vi "Real Cholesky Factorization.vi"(0 "A":T1) -> (1 "Cholesky":T1, 2 "error":i32)   [LabVIEW 2018, in "NI_AALPro.lvlib"]
doc: "Performs Cholesky factorization on a symmetric or Hermitian positive definite matrix. Wire data to the <B>A</B> input to determine the polymorphic instance to use or manually select the instance."
uses:
  <vilib>/Analysis/NI_AALPro.lvlib
  RealMatrix.ctl
  Full Real Matrix Cholesky Factorization.vi
  <vilib>/Analysis/NI_AALBase.lvlib
  NI_Matrix.lvlib
panel:
  # "Cholesky Factorization"
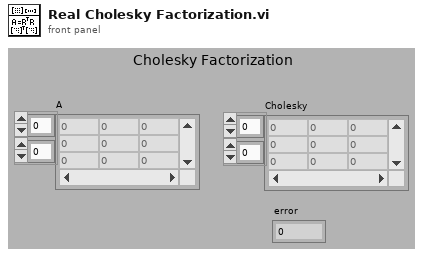
[diagram p1: front panel]
types:
  T1 = typedef "NI_Matrix.lvlib/RealMatrix.ctl" = dbl[][]
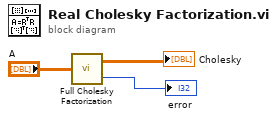
[diagram p0: block diagram]
diagram:
  n1 = call-poly "Full Cholesky Factorization.vi"("A"="A") -> ("Cholesky"=→"Cholesky":T1, "error"=→"error":i32)
